vi "Enqueue Action.vi"(6 "Index in":i64, 10 "Boost in":bool, 11 "Communication in":refnum<class "Communication.lvclass">) -> ()   [LabVIEW 2021, in "Communication.lvclass"]
doc: "MIT Licence\nCopyright (c) 2024 David Grollier"
uses:
  Communication.lvclass
  Communication.lvclass/Communication.ctl
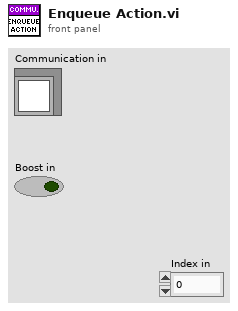
[diagram p1: front panel]
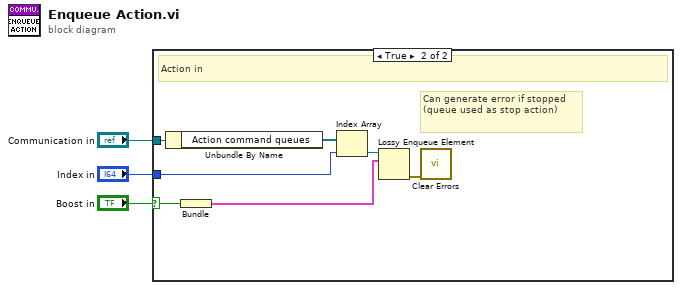
[diagram p0: block diagram]
diagram:
  n1 = case shown="True" "Boost in" {
    selector: "Boost in" -> [_ w6]
    tunnel: "Communication in" -> [_ w8]
    tunnel: "Index in" -> [_ w4]
    frame False {
      # "No action"
    }
    frame True {
      # "Can generate error if stopped (queue used as stop action)"
      # "Action in"
      n2 = Unbundle By Name(w8) -> ("Action command queues"=w7:refnum<queue>[])
      n3 = Bundle(w6) -> (w5:cluster{bool})  [unwired: 1 in]
      n4 = Index Array(array=w7, index=w4) -> (element=w10:refnum<queue>)
      n5 = Lossy Enqueue Element(queue=w10, element=w5) -> (error out=w9:errorcluster)  [unwired: 1 in, 3 out]
      n6 = call <vilib>:"Clear Errors.vi"("error in (no error)"=w9) -> ()  [unwired: 5 in, 2 out]
    }
  }
